vi "Main Page.vi"(8 "error in (no error)":errorcluster, 11 "Node Ptr":T1 format="%.0x") -> (0 "error out":errorcluster)   [LabVIEW 2020, in "Routing and Faulting System Explorer.lvlib"]
uses:
  Routing and Faulting System Explorer.lvlib
  <vilib>/NI VeriStand/Custom Device API/Custom Device Item Ref.ctl
  <vilib>/NI VeriStand/Custom Device API/Custom Device API.lvlib
panel:
  in  "SHDocVw.IWebBrowser":refnum<k7>(container)
types:
  T1 = typedef "Custom Device API.lvlib/Custom Device Item Ref.ctl" = u64
  T2 = typedef "Custom Device API.lvlib/Custom Device Commands.ctl" = enum16{"Default", "Item renamed", "Shutdown", "Dynamic button pressed"}
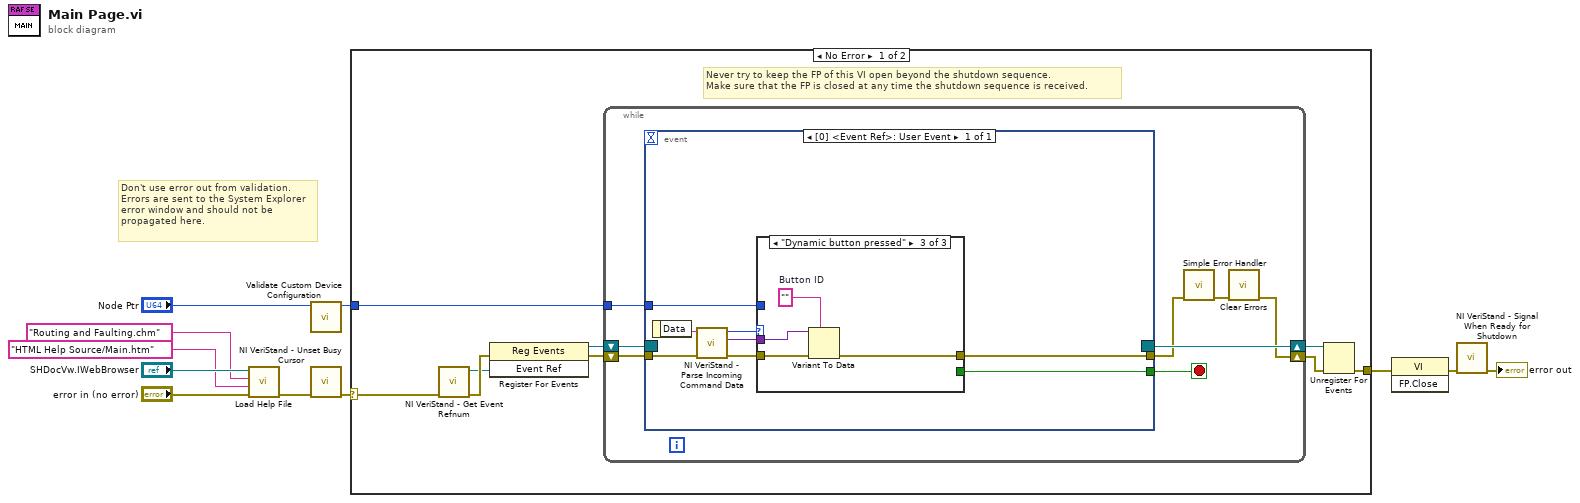
[diagram p0: block diagram]
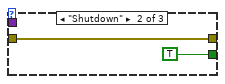
[diagram p3: hidden frame]
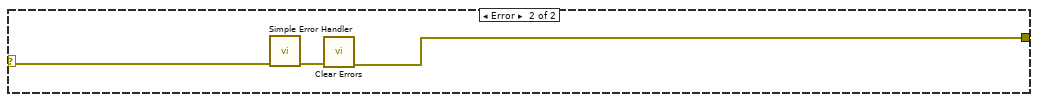
[diagram p4: hidden frame]
diagram:
  # "Don't use error out from validation.\nErrors are sent to the System Explorer\nerror window and should not be\npropagated here."
  n1 = call "Load Help File.vi"("error in (no error)"="error in (no error)", "HTML File to Load"="HTML Help Source/Main.htm" ("HTML File"), "Main CHM File"="Routing and Faulting.chm" ("CD_CHM_FileName"), "Browser"="SHDocVw.IWebBrowser") -> ("error out"=w3:errorcluster)  [unwired: 7 in]
  n2 = call "Validate Custom Device Configuration.vi"("Routing and Faulting Custom Device Ref"="Node Ptr") -> ("Routing and Faulting Custom Device Ref out"=w1:T1)  [unwired: 8 in, 2 out]
  n3 = call <vilib>:"NI VeriStand - Unset Busy Cursor.vi"("error in (no error)"=w3) -> ("error out"=w8:errorcluster)  [unwired: 10 out]
  n4 = case shown="No Error" w8 {
    selector: w8 -> [w13 w46]
    tunnel: [w17 w44] -> w11
    tunnel: w1 -> [w12 _]
    frame No Error {
      # "Never try to keep the FP of this VI open beyond the shutdown sequence.\nMake sure that the FP is closed at any time the shutdown sequence is received."
      n5 = call <vilib>:"NI VeriStand - Get Event Refnum.vi"("error in (no error)"=w13) -> ("error out"=w20:errorcluster, "Event Ref"=w16:refnum<user-event>)  [unwired: 9 out]
      n6 = register-events(error in=w20, w16) -> (reference out=w14:refnum<event-registration>, error out=w15:errorcluster)  [unwired: 1 in]
      n7 = while {
        tunnel: w12 -> [w24]
        shift-right: [w21] -> w18
        shift-left: w15 -> [w27]
        shift-right: [w28] -> w19
        shift-left: w14 -> [w26]
        stop <- w25 stop-if-true
        n8 = event shown="[0] <Event Ref>: User Event" {
          selector: w26 -> [_]
          dyn-events: [_] -> w28
          timeout: _ -> [_]
          tunnel: w27 -> [w36]
          tunnel: [w32] -> w25
          tunnel: [w31] -> w23
          tunnel: w24 -> [w30]
          event User Event {
            n9 = event-data() -> ("Data"=w35:string)  [unwired: 1 out]
            n10 = call <vilib>:"NI VeriStand - Parse Incoming Command Data.vi"("error in (no error)"=w36, "Incoming data"=w35) -> ("error out"=w34:errorcluster, "Outgoing data"=w29:variant, "Action"=w33:T2)  [unwired: 7 out]
            n11 = case shown="\"Dynamic button pressed\"" w33 {
              tunnel: w34 -> [w37 w38 w43]
              tunnel: [_ TRUE _] -> w32
              tunnel: [w37 w38 w40] -> w31
              tunnel: w30 -> [_ _ _]
              tunnel: w29 -> [_ _ w42]
              frame "Default", Default {
              }
              frame "Shutdown" {
              }
              frame "Dynamic button pressed" {
                w41 = ""  # Button ID
                n12 = Variant To Data(error in=w43, type=w41, Variant=w42) -> (error out=w40:errorcluster)  [unwired: 1 out]
              }
            }
          }
        }
        n13 = call <vilib>:"Simple Error Handler.vi"("error in (no error)"=w23) -> ("error out"=w22:errorcluster)  [unwired: 1 in, 7 out]
        n14 = call <vilib>:"Clear Errors.vi"("error in (no error)"=w22) -> ("error out"=w21:errorcluster)  [unwired: 1 in, 5 out]
      }
      n15 = Unregister For Events(event registration refnum=w19, error in=w18) -> (error out=w17:errorcluster)
    }
    frame Error {
      n16 = call <vilib>:"Simple Error Handler.vi"("error in (no error)"=w46) -> ("error out"=w45:errorcluster)  [unwired: 1 in, 7 out]
      n17 = call <vilib>:"Clear Errors.vi"("error in (no error)"=w45) -> ("error out"=w44:errorcluster)  [unwired: 1 in, 5 out]
    }
  }
  n18 = invoke class="VI" method="FP.Close"(error in=w11) -> (error out=w10:errorcluster)  [unwired: 2 in, 2 out]
  n19 = call <vilib>:"NI VeriStand - Signal When Ready for Shutdown.vi"("error in (no error)"=w10) -> ("error out"=→"error out":errorcluster)  [unwired: 10 out]
